vi "Read.vi"   [LabVIEW 2009, in "MicroDAQ.lvlib"]
doc: "Read samples from inputs channels. This VI is polimorphic and will adapt to source."
uses:
  <instrlib>/MicroDAQ/MicroDAQ.lvlib
  <instrlib>/MicroDAQ/Channel/Analog Input/Analog Input.lvclass
  <instrlib>/MicroDAQ/Channel/Digital Input/Digital Input.lvclass
  <instrlib>/MicroDAQ/Channel/DSP/DSP.lvclass
  <instrlib>/MicroDAQ/Channel/Encoder/Encoder.lvclass
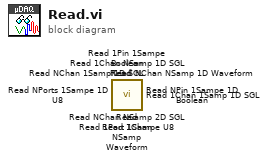
[diagram p0: block diagram]
diagram:
  n1 = call <instrlib>:"Read.vi"() -> ()  [unwired: 8 in, 4 out]
  n2 = call <instrlib>:"Read.vi"() -> ()  [unwired: 9 in, 3 out]
  n3 = call <instrlib>:"Read NPorts 1Sampe 1D U8.vi"() -> ()  [unwired: 9 in, 3 out]
  n4 = call <instrlib>:"Read NPin 1Sampe 1D Boolean.vi"() -> ()  [unwired: 9 in, 3 out]
  n5 = call <instrlib>:"Read 1Port 1Sampe U8.vi"() -> ()  [unwired: 9 in, 3 out]
  n6 = call <instrlib>:"Read 1Pin 1Sampe Boolean.vi"() -> ()  [unwired: 9 in, 3 out]
  n7 = call <instrlib>:"Read NChan NSamp 2D SGL.vi"() -> ()  [unwired: 8 in, 4 out]
  n8 = call <instrlib>:"Read NChan NSamp 1D Waveform.vi"() -> ()  [unwired: 9 in, 3 out]
  n9 = call <instrlib>:"Read NChan 1Samp 1D SGL.vi"() -> ()  [unwired: 9 in, 3 out]
  n10 = call <instrlib>:"Read 1Chan NSamp Waveform.vi"() -> ()  [unwired: 9 in, 3 out]
  n11 = call <instrlib>:"Read 1Chan NSamp 1D SGL.vi"() -> ()  [unwired: 8 in, 4 out]
  n12 = call <instrlib>:"Read 1Chan 1Samp 1D SGL.vi"() -> ()  [unwired: 9 in, 3 out]
